vi "Find Full Custom Channels.vi"(7 "Custom Device Ref":T1 format="%.0x", 8 "error in (no error)":errorcluster, 9 "Channel Descriptors in":T2, 10 "Base path":string, 11 "Full Custom ref":T1 format="%.0x") -> (0 "error out":errorcluster, 1 "Channel Descriptors out":T2)   [LabVIEW 2011, in "Engine Sim System Explorer.lvlib"]
uses:
  Engine Sim System Explorer.lvlib
  <vilib>/NI Veristand/Custom Device API/Custom Device Item Ref.ctl
  Shared/Channel Descriptors.ctl
  Shared/FPGA Write Descriptor.ctl
  Shared/InputChannelTypes.ctl
  <vilib>/rvi/DataTransferAndStorage/Container/Common/niFpgaDataTypeControl.ctl
  Shared/FPGA Read Descriptor.ctl
  Shared/OutputChannelTypes.ctl
  Shared/Status Chan Descriptor.ctl
  <vilib>/NI Veristand/Custom Device Tools/Custom Device Utility Library/NI VeriStand - Search for Item by Name.vi
  <vilib>/NI Veristand/Custom Device Tools/Custom Device Utility Library/Custom Device Utility Library.lvlib
  Engine Simulation Shared.lvlib
  <vilib>/NI Veristand/Custom Device API/Custom Device API.lvlib
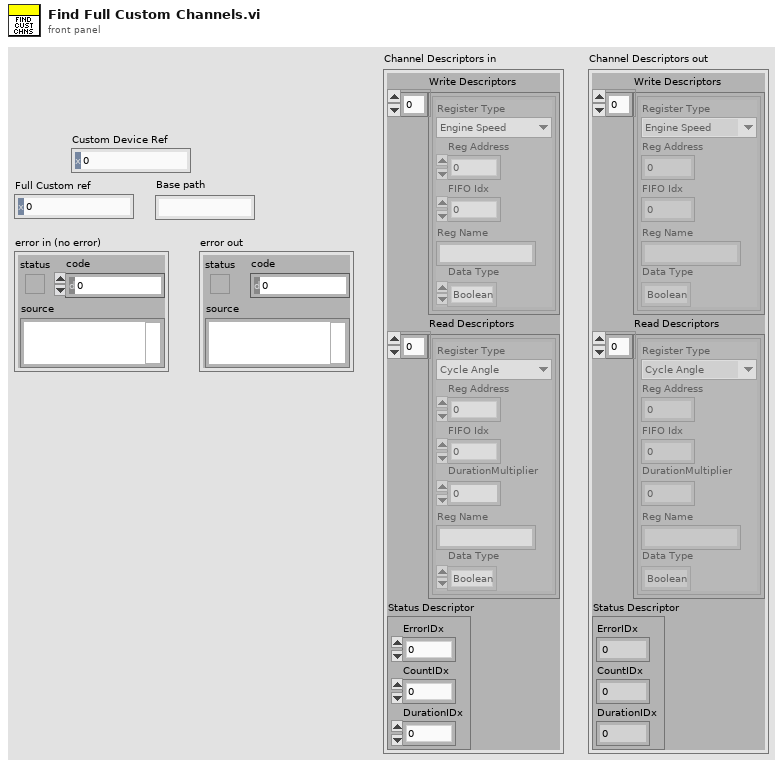
[diagram p1: front panel]
types:
  T1 = typedef "Custom Device API.lvlib/Custom Device Item Ref.ctl" = u64
  T2 = typedef "Engine Simulation Shared.lvlib/Channel Descriptors.ctl" = cluster{"Write Descriptors":T3[], "Read Descriptors":T6[], "Status Descriptor":T8}
  T3 = typedef "Engine Simulation Shared.lvlib/FPGA Write Descriptor.ctl" = cluster{"Register Type":T4, "Reg Address":u32, "FIFO Idx":i32, "Reg Name":string, "Data Type":T5}
  T4 = typedef "Engine Simulation Shared.lvlib/InputChannelTypes.ctl" = enum16{"Engine Speed", "Offset"}
  T5 = typedef "niFpgaDataTypeControl.ctl" = enum32{"Boolean", "I8", "I16", "I32", "I64", "U8", "U16", "U32", "U64", "FXP", "CustomControl"}
  T6 = typedef "Engine Simulation Shared.lvlib/FPGA Read Descriptor.ctl" = cluster{"Register Type":T7, "Reg Address":u32, "FIFO Idx":i32, "DurationMultiplier":dbl, "Reg Name":string, "Data Type":T5}
  T7 = typedef "Engine Simulation Shared.lvlib/OutputChannelTypes.ctl" = enum16{"Cycle Angle", "Crank Angle", "Time Duration", "Angle Duration", "Start Angle", "End Angle"}
  T8 = typedef "Engine Simulation Shared.lvlib/Status Chan Descriptor.ctl" = cluster{"ErrorIDx":i32, "CountIDx":i32, "DurationIDx":i32}
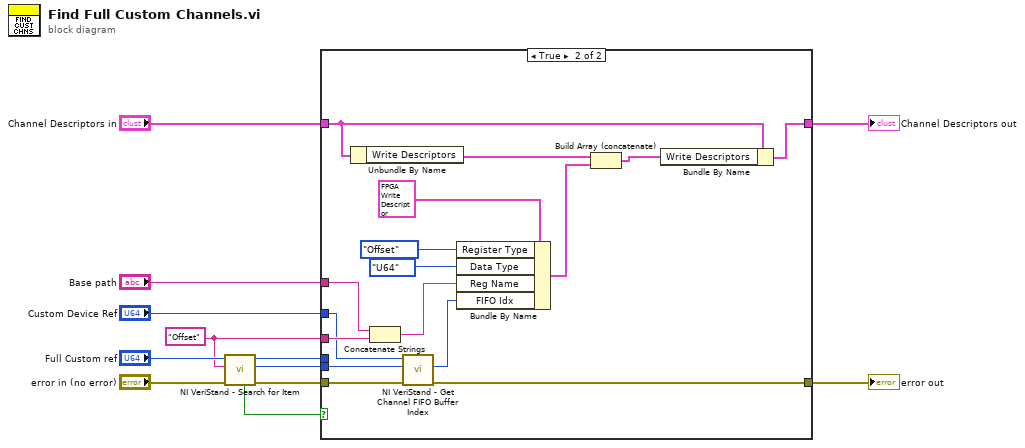
[diagram p0: block diagram]
diagram:
  w6 = "Offset" ("Item Name")
  n1 = call-poly <vilib>:"NI VeriStand - Search for Item.vi"("error in"="error in (no error)", "Item Name"=w6, "Section Ref in"="Full Custom ref") -> ("error out"=w9:errorcluster, "Item Ref"=w8:T1, "Section Ref out"=w1:T1, "Found"=w10:bool)  [unwired: 5 in]
  n2 = case shown="True" w10 {
    tunnel: w9 -> [w13 w22]
    tunnel: w8 -> [_ w21]
    tunnel: "Base path" -> [_ w30]
    tunnel: w6 -> [_ w29]
    tunnel: "Channel Descriptors in" -> [w14 w27]
    tunnel: "Custom Device Ref" -> [_ w20]
    tunnel: [w13 w19] -> w3
    tunnel: [w14 w16] -> w2
    tunnel: w1 -> [_ _]
    frame False {
    }
    frame True {
      n3 = Unbundle By Name(w27) -> ("Write Descriptors"=w28:T3[])
      n4 = Concatenate Strings(w30, w29) -> (w24:string)
      n5 = call <vilib>:"NI VeriStand - Get Channel FIFO Buffer Index.vi"("error in"=w22, "Channel Ref"=w21, "Device Ref in"=w20) -> ("error out"=w19:errorcluster, "Channel FIFO Buffer Index"=w18:i32)  [unwired: 4 in, 3 out]
      n6 = Bundle By Name(cluster=T3 {"Register Type"=enum."Engine Speed", "Reg Address"=0, "FIFO Idx"=0, "Reg Name"="", "Data Type"=enum."Boolean"} ("Write Descriptor"), "Register Type"=InputChannelTypes."Offset", "Data Type"=niFpgaDataTypeControl."U64", "Reg Name"=w24, "FIFO Idx"=w18) -> (w15:T3)
      n7 = Build Array (concatenate)(w28, w15) -> (w17:T3[])
      n8 = Bundle By Name(cluster=w27, "Write Descriptors"=w17) -> (w16:T2)
    }
  }
  "error out" <- w3
  "Channel Descriptors out" <- w2
